vi "Create Plugin Groups.vi"(8 "error in (no error)":errorcluster, 10 "parent tag":string, 11 "Application Data In":T1) -> (0 "error out":errorcluster, 1 "async plugins tag":string, 2 "inline plugins tag":string, 3 "Application Data out":T1)   [LabVIEW 2017, in "DSF Core.lvlib"]
uses:
  DSF Core.lvlib
  Main VI/Application Data.ctl
  <vilib>/NI/Memory Manager/Classes/Pointer/Pointer.lvclass
  Classes/Framework/Framework.lvclass
  Buffer Reader/Buffer Data.ctl
  Classes/Buffer/Buffer.lvclass
  Classes/Transfer Group Status/Transfer Group Status.lvclass
  ID to Tree Items/Tree Item Type.ctl
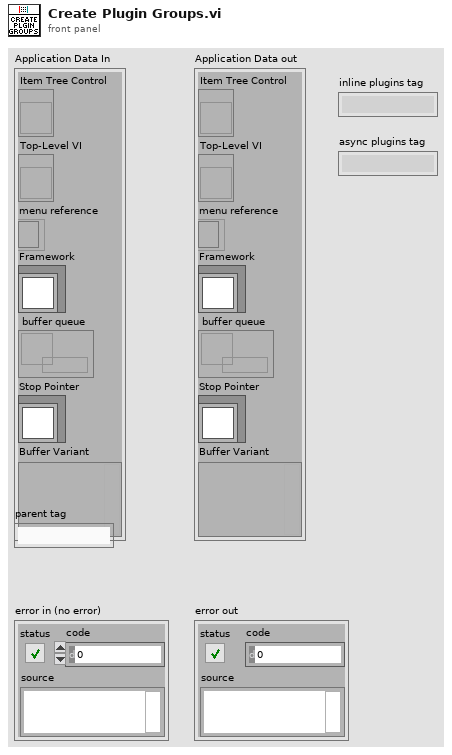
[diagram p1: front panel]
types:
  T1 = typedef "DSF Core.lvlib/Application Data.ctl" = cluster{"Item Tree Control":refnum<vi>, "Top-Level VI":refnum<vi>, "menu reference":refnum<k9>, "Framework":refnum<class "Framework.lvclass">, "buffer queue":refnum<queue>, "Stop Pointer":refnum<class "Pointer.lvclass">, "Buffer Variant":variant}
  T2 = typedef "DSF Core.lvlib/Buffer Data.ctl" = cluster{"Buffer":refnum<class "Buffer.lvclass">, "Status":refnum<class "Transfer Group Status.lvclass">, "decimation":u64, "avg bandwidth":dbl}
  T3 = typedef "DSF Core.lvlib/Tree Item Type.ctl" = enum16{"Framework", "Plugin Group", "Plugin", "Group", "Transfer", "Buffer", "Channel"}
  T4 = typedef "DSF Core.lvlib/Tree Item.ctl" = cluster{"Left Cell String":string, "Child Text":string[], "Child Tag":string, "Glyph Index":i32}
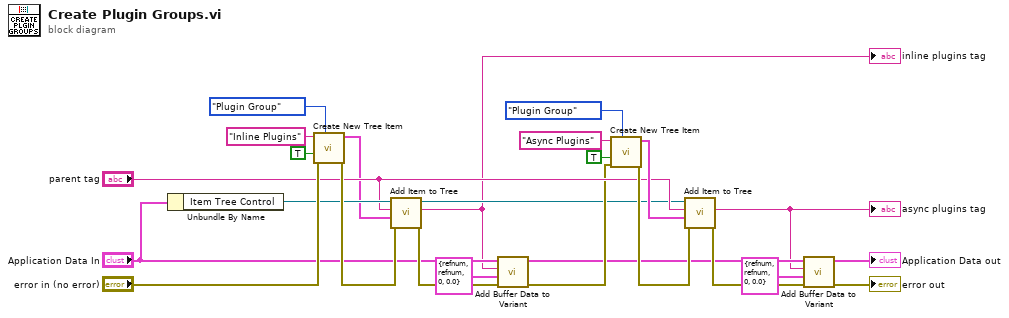
[diagram p0: block diagram]
diagram:
  n1 = Unbundle By Name("Application Data In") -> ("Item Tree Control"=w15:refnum<vi>)
  n2 = call "Create New Tree Item.vi"("Item Type"=Tree_Item_Type."Plugin Group", "error in"="error in (no error)", "found?"=TRUE, "Left Cell String"="Inline Plugins") -> ("error out"=w22:errorcluster, "Item"=w13:T4)  [unwired: 6 in]
  n3 = call "Add Item to Tree.vi"("error in (no error)"=w22, "Item"=w13, "parent tag"="parent tag", "TreeControl in"=w15) -> ("error out"=w11:errorcluster, "new item tag"=w7:string, "TreeControl out"=w8:refnum<vi>)  [unwired: 5 in]
  "inline plugins tag" <- w7
  n4 = call "Add Buffer Data to Variant.vi"("error in (no error)"=w11, "Buffer data"=T2 {"Buffer"=refnum, "Status"=refnum, "decimation"=0, "avg bandwidth"=0.0}, "tag"=w7, "Application Data In in"="Application Data In") -> ("error out"=w12:errorcluster, "Application Data In out"=w2:T1)  [unwired: 6 in]
  n5 = call "Create New Tree Item.vi"("Item Type"=Tree_Item_Type."Plugin Group", "error in"=w12, "found?"=TRUE, "Left Cell String"="Async Plugins") -> ("error out"=w18:errorcluster, "Item"=w17:T4)  [unwired: 6 in]
  n6 = call "Add Item to Tree.vi"("error in (no error)"=w18, "Item"=w17, "parent tag"="parent tag", "TreeControl in"=w8) -> ("error out"=w3:errorcluster, "new item tag"=w1:string)  [unwired: 5 in, 1 out]
  "async plugins tag" <- w1
  n7 = call "Add Buffer Data to Variant.vi"("error in (no error)"=w3, "Buffer data"=T2 {"Buffer"=refnum, "Status"=refnum, "decimation"=0, "avg bandwidth"=0.0}, "tag"=w1, "Application Data In in"=w2) -> ("error out"=→"error out":errorcluster, "Application Data In out"=→"Application Data out":T1)  [unwired: 6 in]
